vi "run state machine.vi"(8 "error in (no error)":errorcluster, 11 "SPARC4_GEI in":refnum<class "SPARC4_GEI.lvclass">) -> (0 "error out":errorcluster, 3 "SPARC4_GEI out":refnum<class "SPARC4_GEI.lvclass">)   [LabVIEW 2018, in "SPARC4_GEI.lvclass"]
uses:
  SPARC4_GEI.lvclass
  SPARC4_GEI.lvclass/SPARC4_GEI.ctl
  Filter_Wheel/Filter_Wheel.lvclass/Filter_Wheel.ctl
  State Machine/State Machine.lvclass/State Machine.ctl
  State Machine/State Machine.lvclass
  TCS/TCS.lvclass
  Channel GUI/Channel GEI.lvclass
  Filter_Wheel/Filter_Wheel.lvclass
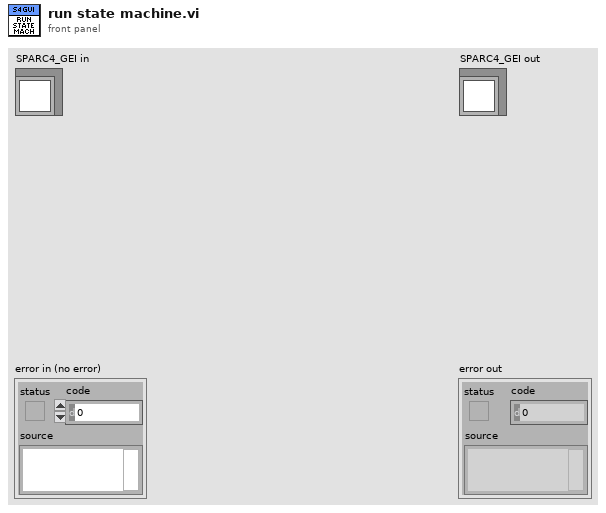
[diagram p1: front panel]
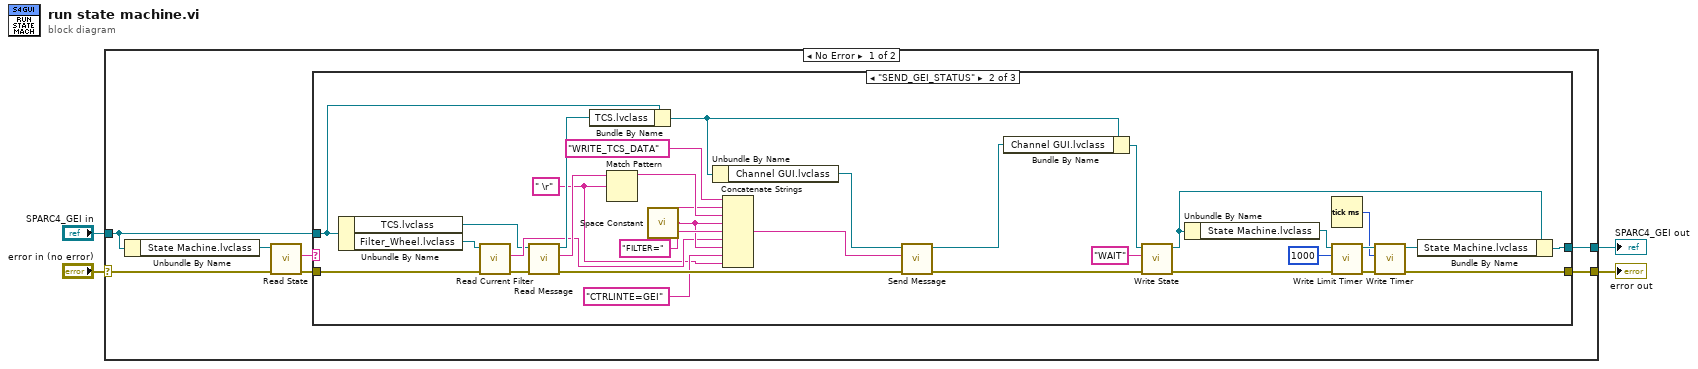
[diagram p0: block diagram]
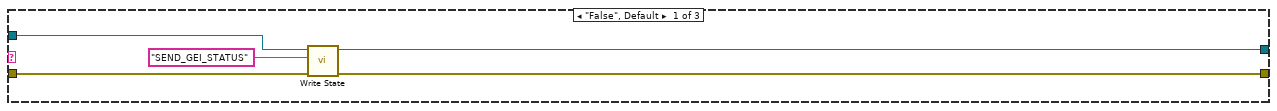
[diagram p2: hidden frame]
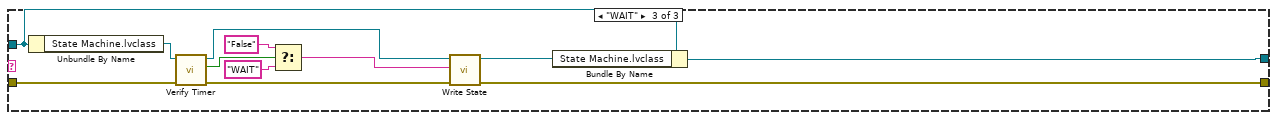
[diagram p3: hidden frame]
diagram:
  n1 = case shown="No Error" "error in (no error)" {
    selector: "error in (no error)" -> [w10 w62]
    tunnel: [w8 w62] -> w3
    tunnel: [w5 w61] -> w1
    tunnel: "SPARC4_GEI in" -> [w6 w61]
    frame No Error {
      n2 = Unbundle By Name(w6) -> ("State Machine.lvclass"=w11:refnum<class "State Machine.lvclass">)
      n3 = call-dynamic "Read State.vi"("error in (no error)"=w10, "State Machine in"=w11) -> ("error out"=w9:errorcluster, "State"=w7:string)  [unwired: 7 in, 1 out]
      n4 = case shown="\"SEND_GEI_STATUS\"" w7 {
        tunnel: w9 -> [w12 w33 w57]
        tunnel: [w14 w23 w55] -> w8
        tunnel: [w15 w26 w60] -> w5
        tunnel: w6 -> [w13 w32 w59]
        frame "False", Default {
          n5 = call "Write State.vi"("error in (no error)"=w12, "State"="SEND_GEI_STATUS", "SPARC4_GEI in"=w13) -> ("error out"=w14:errorcluster, "SPARC4_GEI out"=w15:refnum<class "SPARC4_GEI.lvclass">)  [unwired: 7 in]
        }
        frame "SEND_GEI_STATUS" {
          w17 = " \r" ("regular expression")
          n6 = Unbundle By Name(w32) -> ("TCS.lvclass"=w35:refnum<class "TCS.lvclass">, "Filter_Wheel.lvclass"=w34:refnum<class "Filter_Wheel.lvclass">)
          n7 = call "Read Current Filter.vi"("error in (no error)"=w33, "Filter_Wheel in"=w34) -> ("error out"=w37:errorcluster, "Current Filter"=w36:string)  [unwired: 7 in, 1 out]
          n8 = call "Read Message.vi"("error in (no error)"=w37, "TCS in"=w35) -> ("error out"=w46:errorcluster, "Rx Message"=w41:string, "TCS out"=w47:refnum<class "TCS.lvclass">)  [unwired: 7 in]
          n9 = Bundle By Name(cluster=w32, "TCS.lvclass"=w47) -> (w29:refnum<class "SPARC4_GEI.lvclass">)
          n10 = Match Pattern(string=w41, regular expression=w17) -> (before substring=w40:string)  [unwired: 1 in, 3 out]
          n11 = call <vilib>:"Space Constant.vi"() -> ("String"=w39:string)
          n12 = Unbundle By Name(w29) -> ("Channel GUI.lvclass"=w48:refnum<class "Channel GEI.lvclass">)
          n13 = Concatenate Strings("WRITE_TCS_DATA", w39, w40, w39, "FILTER=", w36, w39, "CTRLINTE=GEI", w17) -> (w44:string)
          n14 = call "Send Message.vi"("error in (no error)"=w46, "Message"=w44, "Channel GUI in"=w48) -> ("error out"=w30:errorcluster, "Channel GUI out"=w45:refnum<class "Channel GEI.lvclass">)  [unwired: 7 in]
          n15 = Bundle By Name(cluster=w29, "Channel GUI.lvclass"=w45) -> (w31:refnum<class "SPARC4_GEI.lvclass">)
          n16 = call "Write State.vi"("error in (no error)"=w30, "State"="WAIT", "SPARC4_GEI in"=w31) -> ("error out"=w21:errorcluster, "SPARC4_GEI out"=w27:refnum<class "SPARC4_GEI.lvclass">)  [unwired: 7 in]
          n17 = Unbundle By Name(w27) -> ("State Machine.lvclass"=w20:refnum<class "State Machine.lvclass">)
          n18 = Tick Count (ms)() -> (millisecond timer value=w18:u32)
          n19 = call "Write Limit Timer.vi"("error in (no error)"=w21, "Limit Timer"=u32 1000, "State Machine in"=w20) -> ("error out"=w22:errorcluster, "State Machine out"=w25:refnum<class "State Machine.lvclass">)  [unwired: 7 in]
          n20 = call "Write Timer.vi"("error in (no error)"=w22, "Timer"=w18, "State Machine in"=w25) -> ("error out"=w23:errorcluster, "State Machine out"=w24:refnum<class "State Machine.lvclass">)  [unwired: 7 in]
          n21 = Bundle By Name(cluster=w27, "State Machine.lvclass"=w24) -> (w26:refnum<class "SPARC4_GEI.lvclass">)
        }
        frame "WAIT" {
          n22 = Unbundle By Name(w59) -> ("State Machine.lvclass"=w58:refnum<class "State Machine.lvclass">)
          n23 = call "Verify Timer.vi"("error in (no error)"=w57, "State Machine in"=w58) -> ("error out"=w51:errorcluster, "time out"=w54:bool, "State Machine out"=w52:refnum<class "State Machine.lvclass">)  [unwired: 7 in]
          n24 = Select(t="False", s=w54, f="WAIT") -> (s? t:f=w53:string)
          n25 = call-dynamic "Write State.vi"("error in (no error)"=w51, "State"=w53, "State Machine in"=w52) -> ("error out"=w55:errorcluster, "State Machine out"=w56:refnum<class "State Machine.lvclass">)  [unwired: 7 in]
          n26 = Bundle By Name(cluster=w59, "State Machine.lvclass"=w56) -> (w60:refnum<class "SPARC4_GEI.lvclass">)
        }
      }
    }
    frame Error {
    }
  }
  "error out" <- w3
  "SPARC4_GEI out" <- w1
